vi "Get Last Row Index.vi"(8 "error in":errorcluster, 11 "Worksheet in":refnum<k24>) -> (0 "error out":errorcluster, 2 "Highest Row Index":u32, 3 "Worksheet out":refnum<k24>)   [LabVIEW 2019, in "Open Xml.lvlib"]
uses:
  Open Xml.lvlib
  D:/git/Open-Xml-LabVIEW/Source/DocumentFormat.OpenXml.dll
  DocumentFormat.OpenXml.dll
  D:/git/Open-Xml-LabVIEW/Source/DocumentFormat.OpenXml.Framework.dll
  DocumentFormat.OpenXml.Framework.dll
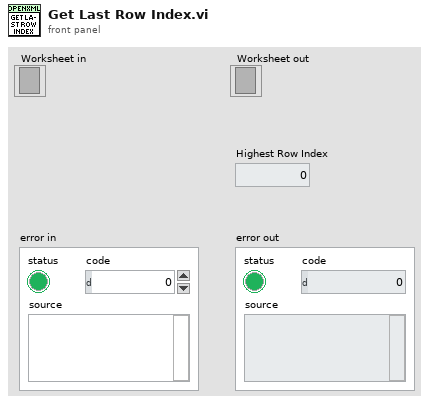
[diagram p1: front panel]
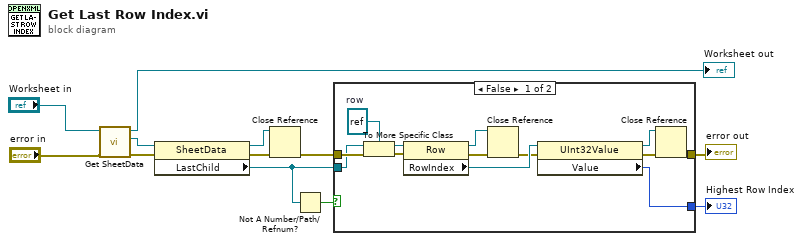
[diagram p0: block diagram]
diagram:
  n1 = call "Get SheetData.vi"("error in"="error in", "Worksheet in"="Worksheet in") -> ("error out"=w10:errorcluster, "SheetData"=w8:refnum<k24>, "Worksheet out"=→"Worksheet out":refnum<k24>)  [unwired: 7 in]
  n2 = property class="SheetData"(reference=w8, error in=w10) -> (reference out=w6:refnum<k24>, error out=w9:errorcluster, "LastChild"=w2:refnum<k24>)
  n3 = Close Reference(reference=w6, error in (no error)=w9) -> (error out=w7:errorcluster)
  n4 = Not A Number/Path/Refnum?(number/path/refnum=w2) -> (NaN/Path/Refnum?=w1:bool)
  n5 = case shown="False" w1 {
    tunnel: w7 -> [w24 w26]
    tunnel: [w17 _] -> w4
    tunnel: [w14 w26] -> w3
    tunnel: w2 -> [w13 _]
    frame False {
      w25 = refnum<k24> refnum  # row
      n6 = To More Specific Class(target class=w25, reference=w13, error in=w24) -> (specific class reference=w22:refnum<k24>, error out=w23:errorcluster)
      n7 = property class="Row"(reference=w22, error in=w23) -> (reference out=w20:refnum<k24>, error out=w19:errorcluster, "RowIndex"=w21:refnum<k24>)
      n8 = Close Reference(reference=w20, error in (no error)=w19) -> (error out=w18:errorcluster)
      n9 = property class="UInt32Value"(reference=w21, error in=w18) -> (reference out=w15:refnum<k24>, error out=w16:errorcluster, "Value"=w17:u32)
      n10 = Close Reference(reference=w15, error in (no error)=w16) -> (error out=w14:errorcluster)
    }
    frame True {
    }
  }
  "error out" <- w3
  "Highest Row Index" <- w4
